vi "Pre Launch Init.vi"(11 "Engine_Tools in":refnum<class "Engine.lvclass">) -> (0 "error out":errorcluster, 3 "Engine_Tools out":refnum<class "Engine.lvclass">)   [LabVIEW 2019, in "Engine.lvlib" / "Engine.lvclass"]
doc: "This routine determines if the instance calling the function is the root actor. \n<b>Root Actor </b> reads its self-enqueuer in to private data\n\n<b>Nested Actor</b> reads its self-enqueuer and the caller enqueuer in to private data"
uses:
  Project/Engine.lvclass
  builds/Engine/State Actor.lvlibp/Library/State Actor.lvclass
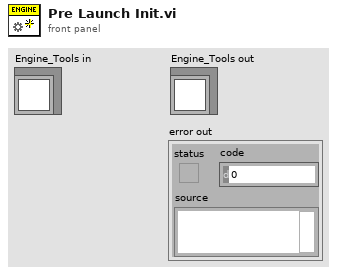
[diagram p1: front panel]
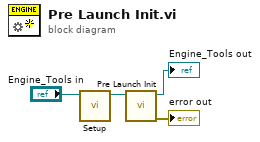
[diagram p0: block diagram]
diagram:
  n1 = call "Setup.vi"("Fault_Engine in"="Engine_Tools in") -> ("Fault_Engine out"=w1:refnum<class "Engine.lvclass">)  [unwired: 9 in, 1 out]
  n2 = call-parent "Pre Launch Init.vi"("Panel Actor in"=w1) -> ("error out"=→"error out":errorcluster, "Panel Actor out"=→"Engine_Tools out":refnum<class "Engine.lvclass">)  [unwired: 9 in]
